vi "DCM Core Interface.vi"(6 "Device Inputs":dbl[](array[numeric]), 8 "error in":errorcluster, 9 "Device Outputs in":dbl[](array[numeric]), 10 "DCM Ref":refnum<class "DCM - RT.lvclass">, 11 "DCM Core in":T1={"FIFO Indexes"={"A Run State"=-1, "B Run State"=-1, "Read"={"Status"={"System ADC"={"AI 1 [V]"=0, "AI 2 [V]"=0, "AI 3 [V]"=0, "AI 4 [V]"=0, "AI 5 [V]"=0, "AI 6 [V]"=0, "AI 7 [V]"=0, "AI 8 [V]"=0, "AI 9 [V]"=0, "AI 10 [V]"=0, "AI 11 [V]"=0, "AI 12 [V]"=0, "Temp HH 1-6 [C]"=0, "Temp HH 7-12 [C]"=0, "Temp DI A [C]"=0, "Temp DI Zener A [C]"=0, "Temp DI B [C]"=0, "Temp DI Zener B [C]"=0, "Temp CPU [C]"=0, "Temp Fan Intake [C]"=0, "Temp Secondary A [C]"=0, "Temp Primary A [C]"=0, "Temp Boost B [C]"=0, "Primary Range [V]"=0, "Primary A1A2 [V]"=0, "Primary A3A4 [V]"=0, "Primary B3B4 [V]"=0, "Primary B1B2 [V]"=0, "Secondary A1A2 [V]"=0, "Secondary A3A4 [V]"=0, "Secondary B3B4 [V]"=0, "Secondary B1B2 [V]"=0, "Ext HV A [V]"=0, "Ext HV B [V]"=0, "FET Driver [V]"=0, "Fan [V]"=-1, "Battery [V]"=0, "DRVP [V]"=0, "Key [V]"=0, "DI Zener A [V]"=0, "DI Zener B [V]"=0, "Pump Zener A [V]"=0, "Pump Zener B [V]"=0, "MPRD [V]"=0}, "IO Lock"=0, "HH Mode Config Error"=0, "Fan Speed 1 [RPM]"=0, "Fan Speed 2 [RPM]"=0, "Firmware Major Rev"=0, "Firmware Minor Rev"=0, "Internal Fault"=-1, "Fault Value"=-1}, "A DI Faults"=[], "B DI Faults"=[], "HH Status"=[]}, "Write"={"A Config"={"PowerSupplyEnable"=0, "InjectEnable"=0, "BoostVoltage"=0}, "B Config"={"PowerSupplyEnable"=0, "InjectEnable"=0, "BoostVoltage"=0}, "HH Config"=[], "System Settings"={"MPRD"=0, "UserLED1"=0, "UserLED2"=0}, "A Fault Clear"={"1"=0, "2"=0, "3"=0, "4"=0, "5"=0, "6"=0, "7"=0, "8"=0}, "B Fault Clear"={"1"=0, "2"=0, "3"=0, "4"=0, "5"=0, "6"=0, "7"=0, "8"=0}}}, "Settings"={"A Configuration"={"Configuration"=enum."Solenoid Unipolar 4", "Power Supply Enable"=FALSE, "Boost Voltage [V]"=0.0, "Inject Enable"=FALSE, "DI Zener Enable"=FALSE, "DI Zener Voltage [V]"=0.0, "Pump Zener Enable"=FALSE, "Pump Zener Voltage [V]"=0.0, "Boost Clamp [V]"=0.0}, "B Configuration"={"Configuration"=enum."Solenoid Unipolar 4", "Power Supply Enable"=FALSE, "Boost Voltage [V]"=0.0, "Inject Enable"=FALSE, "DI Zener Enable"=FALSE, "DI Zener Voltage [V]"=0.0, "Pump Zener Enable"=FALSE, "Pump Zener Voltage [V]"=0.0, "Boost Clamp [V]"=0.0}, "System Settings"={"MPRD"=FALSE, "IO Lock MPRD Disable"=FALSE, "User LED 1"=enum."Off", "User LED 2"=enum."Off", "DI HS Fault Filter Time [s]"=0.0, "Clamp Fault Filter Time [s]"=0.0, "HH Shoot Through Time [s]"=0.0, "HH ISeq Dur PS"=0, "HH Open Threshold [A]"=0.0}}} {"Settings"."System Settings"."HH Open Threshold [A]" min=0 max=8 format="%#_3p"; "Settings"."System Settings"."HH ISeq Dur PS" items=["3.3ms @ 20MHz"=0, "6.5ms @ 10MHz"=4, "13ms @ 5MHz"=6, "26ms @ 2.5MHz"=7]; "Settings"."System Settings"."HH Shoot Through Time [s]" min=0 max=0.003277 format="%#_3p"; "Settings"."System Settings"."Clamp Fault Filter Time [s]" min=0 max=0.003277 format="%#_3p"; "Settings"."System Settings"."DI HS Fault Filter Time [s]" min=0 max=0.003277 format="%#_3p"; "Settings"."B Configuration"."Pump Zener Voltage [V]" min=0 max=240 format="%#_13g"; "Settings"."B Configuration"."DI Zener Voltage [V]" min=0 max=100 format="%#_13g"; "Settings"."B Configuration"."Boost Clamp [V]" min=0 max=220 format="%#_13g"; "Settings"."B Configuration"."Boost Voltage [V]" min=0 max=220 format="%#_13g"; "Settings"."A Configuration"."Pump Zener Voltage [V]" min=0 max=240 format="%#_13g"; "Settings"."A Configuration"."DI Zener Voltage [V]" min=0 max=100 format="%#_13g"; "Settings"."A Configuration"."Boost Clamp [V]" min=0 max=220 format="%#_13g"; "Settings"."A Configuration"."Boost Voltage [V]" min=0 max=220 format="%#_13g"; "FIFO Indexes"."Write"."HH Config"."ISeq"."Duration [s]" min=0 max=26; "FIFO Indexes"."Write"."HH Config"."ISeq"."Lower [A]" min=0 max=8; "FIFO Indexes"."Write"."HH Config"."ISeq"."Upper [A]" min=0 max=8}) -> (0 "error out":errorcluster, 1 "Device Outputs out":dbl[](array[numeric]))   [LabVIEW 2016, in "DCM Engine.lvlib"]
uses:
  DCM Engine.lvlib
  Shared/Types/DCM Core.ctl
  Shared/Types/System State Indexes.ctl
  Shared/Types/DI Faults Indexes.ctl
  Shared/Types/HH Status Indexes.ctl
  Shared/Types/HH Config Indexes.ctl
  <vilib>/Powertrain Controls/Device Drivers/DCM/Rev0/RT/Configuration.ctl
  <vilib>/Powertrain Controls/Device Drivers/DCM/Rev0/FPGA/DI - Bank Configuration.ctl
  <vilib>/Powertrain Controls/Device Drivers/DCM/Rev0/RT/System Settings.ctl
  <vilib>/Powertrain Controls/Device Drivers/DCM/Rev0/RT/User LED.ctl
  <vilib>/Powertrain Controls/Device Drivers/DCM/HH/RT/Duration Pre Scale.ctl
  Built/DCM Classes Packed/Pharlap/C/DCM-Classes.lvlibp/DCM/Rev0/RT/DCM - RT.lvclass
  DCM Shared.lvlib
  <vilib>/Powertrain Controls/Device Drivers/DCM/Rev0/RT/DCM - RT.lvclass
  <vilib>/Powertrain Controls/Device Drivers/DCM/Rev0/FPGA/DCM - FPGA.lvlib
  <vilib>/Powertrain Controls/Device Drivers/DCM/HH/RT/DCM - RT - HH.lvlib
panel:
  # "Voltage [DV]"
  # "Voltage [V]"
  # "Voltage [DV]"
  # "Voltage [V]"
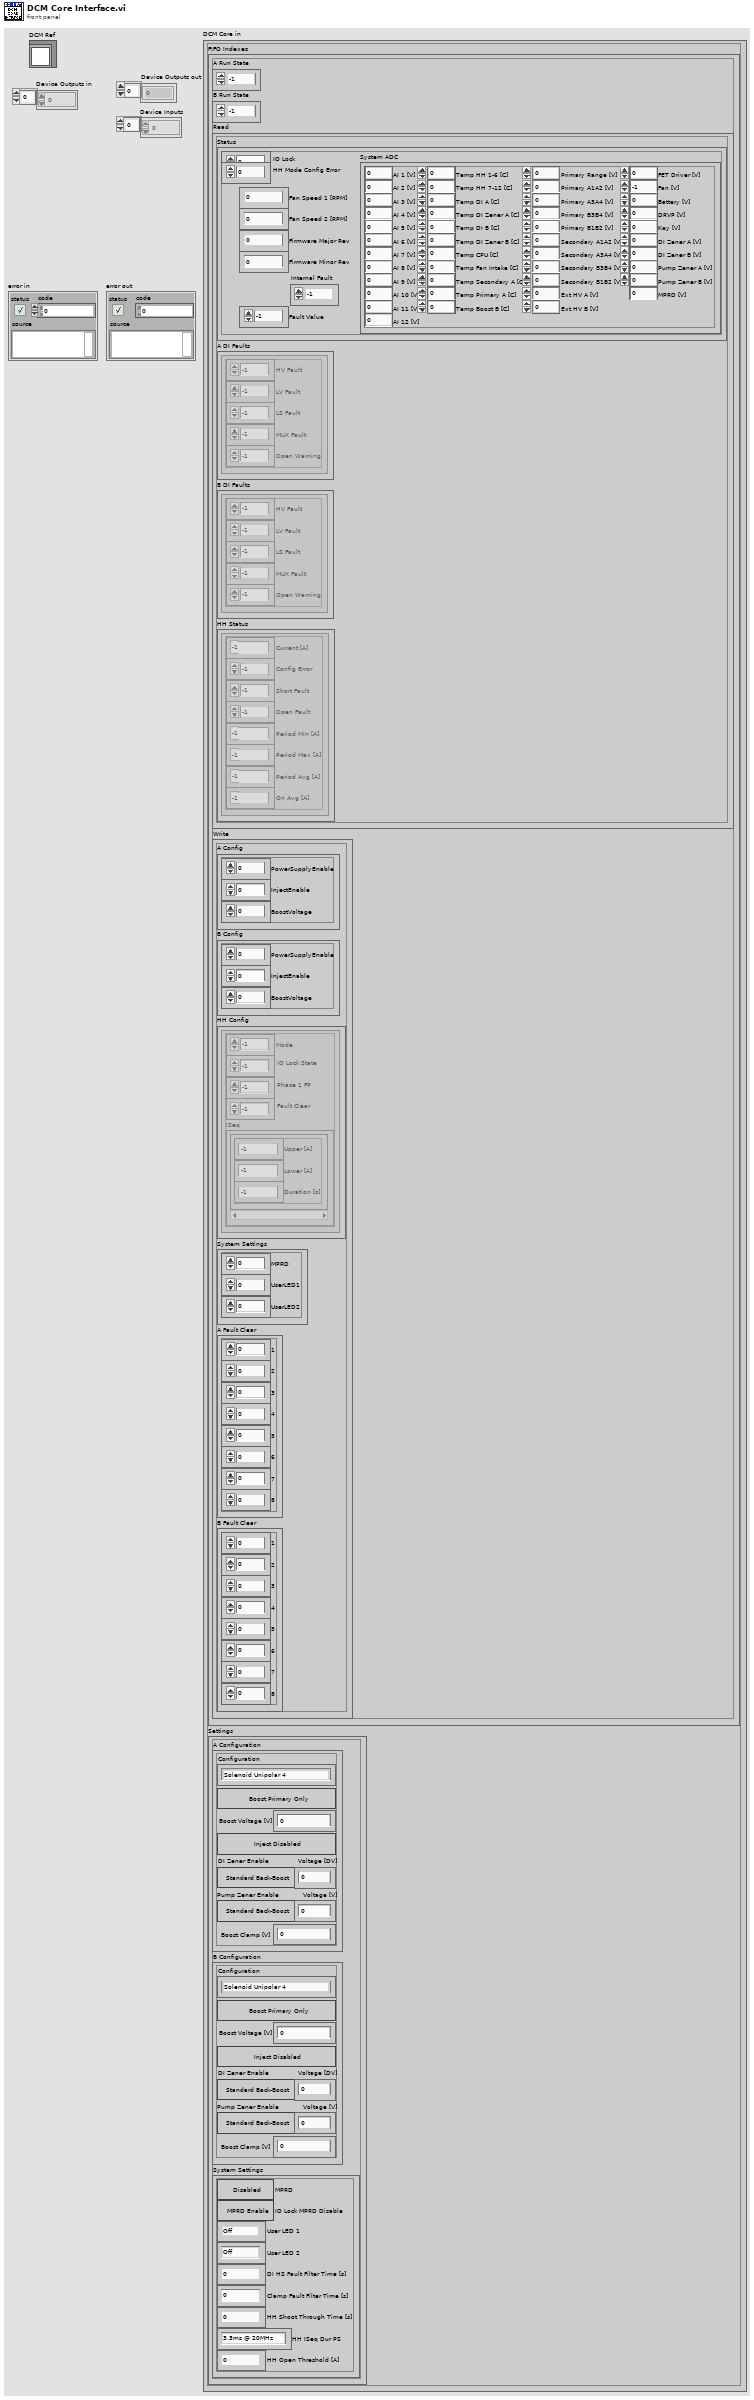
[diagram p1: front panel]
types:
  T1 = typedef "DCM Shared.lvlib/DCM Core.ctl" = cluster{"FIFO Indexes":cluster{"A Run State":i32, "B Run State":i32, "Read":cluster{"Status":T2, "A DI Faults":T3[], "B DI Faults":T3[], "HH Status":T4[]}, "Write":cluster{"A Config":cluster{"PowerSupplyEnable":i32, "InjectEnable":i32, "BoostVoltage":i32}, "B Config":cluster{"PowerSupplyEnable":i32, "InjectEnable":i32, "BoostVoltage":i32}, "HH Config":T5[], "System Settings":cluster{"MPRD":i32, "UserLED1":i32, "UserLED2":i32}, "A Fault Clear":cluster{"1":i32, "2":i32, "3":i32, "4":i32, "5":i32, "6":i32, "7":i32, "8":i32}, "B Fault Clear":cluster{"1":i32, "2":i32, "3":i32, "4":i32, "5":i32, "6":i32, "7":i32, "8":i32}}}, "Settings":cluster{"A Configuration":T6, "B Configuration":T6, "System Settings":T8}}
  T2 = typedef "DCM Shared.lvlib/System State Indexes.ctl" = cluster{"System ADC":cluster{"AI 1 [V]":i32, "AI 2 [V]":i32, "AI 3 [V]":i32, "AI 4 [V]":i32, "AI 5 [V]":i32, "AI 6 [V]":i32, "AI 7 [V]":i32, "AI 8 [V]":i32, "AI 9 [V]":i32, "AI 10 [V]":i32, "AI 11 [V]":i32, "AI 12 [V]":i32, "Temp HH 1-6 [C]":i32, "Temp HH 7-12 [C]":i32, "Temp DI A [C]":i32, "Temp DI Zener A [C]":i32, "Temp DI B [C]":i32, "Temp DI Zener B [C]":i32, "Temp CPU [C]":i32, "Temp Fan Intake [C]":i32, "Temp Secondary A [C]":i32, "Temp Primary A [C]":i32, "Temp Boost B [C]":i32, "Primary Range [V]":i32, "Primary A1A2 [V]":i32, "Primary A3A4 [V]":i32, "Primary B3B4 [V]":i32, "Primary B1B2 [V]":i32, "Secondary A1A2 [V]":i32, "Secondary A3A4 [V]":i32, "Secondary B3B4 [V]":i32, "Secondary B1B2 [V]":i32, "Ext HV A [V]":i32, "Ext HV B [V]":i32, "FET Driver [V]":i32, "Fan [V]":i32, "Battery [V]":i32, "DRVP [V]":i32, "Key [V]":i32, "DI Zener A [V]":i32, "DI Zener B [V]":i32, "Pump Zener A [V]":i32, "Pump Zener B [V]":i32, "MPRD [V]":i32}, "IO Lock":i32, "HH Mode Config Error":i32, "Fan Speed 1 [RPM]":i32, "Fan Speed 2 [RPM]":i32, "Firmware Major Rev":i32, "Firmware Minor Rev":i32, "Internal Fault":i32, "Fault Value":i32}
  T3 = typedef "DCM Shared.lvlib/DI Faults Indexes.ctl" = cluster{"HV Fault":i32, "LV Fault":i32, "LS Fault":i32, "MUX Fault":i32, "Open Warning":i32}
  T4 = typedef "DCM Shared.lvlib/HH Status Indexes.ctl" = cluster{"Current [A]":i32, "Config Error":i32, "Short Fault":i32, "Open Fault":i32, "Period Min [A]":i32, "Period Max [A]":i32, "Period Avg [A]":i32, "On Avg [A]":i32}
  T5 = typedef "DCM Shared.lvlib/HH Config Indexes.ctl" = cluster{"Mode":i32, "IO Lock State":i32, "Phase 1 FP":i32, "Fault Clear":i32, "ISeq":cluster{"Upper [A]":i32, "Lower [A]":i32, "Duration [s]":i32}[]}
  T6 = typedef "DCM - RT.lvclass/Configuration.ctl" = cluster{"Configuration":T7, "Power Supply Enable":bool, "Boost Voltage [V]":sgl, "Inject Enable":bool, "DI Zener Enable":bool, "DI Zener Voltage [V]":sgl, "Pump Zener Enable":bool, "Pump Zener Voltage [V]":sgl, "Boost Clamp [V]":sgl}
  T7 = typedef "DCM - FPGA.lvlib/DI - Bank Configuration.ctl" = enum8{"Solenoid Unipolar 4", "Solenoid Unipolar 7 (Muxed)", "Solenoid Unipolar 8 (Muxed)", "Solenoid Bipolar 2", "Solenoid Bipolar 3 (Muxed)", "Piezo Unipolar 2", "Piezo Unipolar 3 (Muxed)", "Piezo Unipolar 4 (Muxed)", "Piezo Bipolar 2", "Piezo Bipolar 3 (Muxed)"}
  T8 = typedef "DCM - RT.lvclass/System Settings.ctl" = cluster{"MPRD":bool, "IO Lock MPRD Disable":bool, "User LED 1":T9, "User LED 2":T9, "DI HS Fault Filter Time [s]":sgl, "Clamp Fault Filter Time [s]":sgl, "HH Shoot Through Time [s]":sgl, "HH ISeq Dur PS":T10, "HH Open Threshold [A]":sgl}
  T9 = typedef "DCM - RT.lvclass/User LED.ctl" = enum16{"Off", "Yellow", "Green"}
  T10 = typedef "DCM - RT - HH.lvlib/Duration Pre Scale.ctl" = u8
  T11 = typedef "DCM-Classes.lvlibp/DCM - RT.lvclass/System Settings.ctl" = cluster{"MPRD":bool, "IO Lock MPRD Disable":bool, "User LED 1":T12, "User LED 2":T12, "DI HS Fault Filter Time [s]":sgl, "Clamp Fault Filter Time [s]":sgl, "HH Shoot Through Time [s]":sgl, "HH ISeq Dur PS":T13, "HH Open Threshold [A]":sgl}
  T12 = typedef "DCM-Classes.lvlibp/DCM - RT.lvclass/User LED.ctl" = enum16{"Off", "Yellow", "Green"}
  T13 = typedef "DCM-Classes.lvlibp/DCM - RT - HH.lvlib/Duration Pre Scale.ctl" = u8
  T14 = typedef "DCM-Classes.lvlibp/DCM - RT.lvclass/Configuration.ctl" = cluster{"Configuration":T15, "Power Supply Enable":bool, "Boost Voltage [V]":sgl, "Inject Enable":bool, "DI Zener Enable":bool, "DI Zener Voltage [V]":sgl, "Pump Zener Enable":bool, "Pump Zener Voltage [V]":sgl, "Boost Clamp [V]":sgl}
  T15 = typedef "DCM-Classes.lvlibp/DCM - FPGA.lvlib/DI - Bank Configuration.ctl" = enum8{"Solenoid Unipolar 4", "Solenoid Unipolar 7 (Muxed)", "Solenoid Unipolar 8 (Muxed)", "Solenoid Bipolar 2", "Solenoid Bipolar 3 (Muxed)", "Piezo Unipolar 2", "Piezo Unipolar 3 (Muxed)", "Piezo Unipolar 4 (Muxed)", "Piezo Bipolar 2", "Piezo Bipolar 3 (Muxed)"}
  T16 = typedef "DCM - FPGA - Tools.lvlib/8 Channels.ctl" = cluster{"1":bool, "2":bool, "3":bool, "4":bool, "5":bool, "6":bool, "7":bool, "8":bool}
  T17 = typedef "DCM-Classes.lvlibp/DCM - RT - HH.lvlib/Config.ctl" = cluster{"Mode":T18, "IO Lock State":bool, "Phase 1 FP":bool, "Fault Clear":bool, "ISeq":T19[]}
  T18 = typedef "DCM-Classes.lvlibp/DCM - RT - HH.lvlib/Mode.ctl" = enum16{"Off", "Lowside", "Highside", "PFI", "Full H", "3-Phase"}
  T19 = typedef "DCM-Classes.lvlibp/DCM - RT - HH.lvlib/ISeq.ctl" = cluster{"Upper [A]":sgl, "Lower [A]":sgl, "Duration [s]":sgl}
  T20 = typedef "DCM-Classes.lvlibp/DCM - RT.lvclass/Run State.ctl" = enum8{"Idle", "Warmup", "Ready To Inject", "Cool Down"}
  T21 = typedef "DCM-Classes.lvlibp/DCM - RT.lvclass/System State.ctl" = cluster{"System ADC":T22, "IO Lock":bool, "HH Mode Config Error":bool, "Fan Speed 1 [RPM]":sgl, "Fan Speed 2 [RPM]":sgl, "Firmware Major Rev":u16, "Firmware Minor Rev":u16, "Internal Fault":T23, "Fault Value":dbl}
  T22 = typedef "DCM-Classes.lvlibp/DCM - RT.lvclass/System ADC.ctl" = cluster{"AI 1 [V]":sgl, "AI 2 [V]":sgl, "AI 3 [V]":sgl, "AI 4 [V]":sgl, "AI 5 [V]":sgl, "AI 6 [V]":sgl, "AI 7 [V]":sgl, "AI 8 [V]":sgl, "AI 9 [V]":sgl, "AI 10 [V]":sgl, "AI 11 [V]":sgl, "AI 12 [V]":sgl, "Temp HH 1-6 [C]":sgl, "Temp HH 7-12 [C]":sgl, "Temp DI A [C]":sgl, "Temp DI Zener A [C]":sgl, "Temp DI B [C]":sgl, "Temp DI Zener B [C]":sgl, "Temp CPU [C]":sgl, "Temp Fan Intake [C]":sgl, "Temp Secondary A [C]":sgl, "Temp Primary A [C]":sgl, "Temp Boost B [C]":sgl, "Primary Range [V]":sgl, "Primary A1A2 [V]":sgl, "Primary A3A4 [V]":sgl, "Primary B3B4 [V]":sgl, "Primary B1B2 [V]":sgl, "Secondary A1A2 [V]":sgl, "Secondary A3A4 [V]":sgl, "Secondary B3B4 [V]":sgl, "Secondary B1B2 [V]":sgl, "Ext HV A [V]":sgl, "Ext HV B [V]":sgl, "FET Driver [V]":sgl, "Fan [V]":sgl, "Battery [V]":sgl, "DRVP [V]":sgl, "Key [V]":sgl, "DI Zener A [V]":sgl, "DI Zener B [V]":sgl, "Pump Zener A [V]":sgl, "Pump Zener B [V]":sgl, "MPRD [V]":sgl}
  T23 = typedef "DCM-Classes.lvlibp/DCM - RT.lvclass/Internal Fault.ctl" = enum32{"None", "Temp HH 1-6", "Temp HH 7-12", "Temp DI A", "Temp DI Zener A", "Temp DI B", "Temp DI Zener B", "Temp Intake", "Temp Primary A", "Temp Secondary A", "Temp Boost B", "Temp CPU", "Low Battery", "Inrush Protection", "A Run Enable", "B Run Enable"}
  T24 = typedef "DCM-Classes.lvlibp/DCM - FPGA.lvlib/DI - Faults.ctl" = cluster{"HV Fault":bool, "LV Fault":bool, "LS Fault":bool, "MUX Fault":bool, "Open Warning":bool}
  T25 = typedef "DCM-Classes.lvlibp/DCM - RT - HH.lvlib/Status.ctl" = cluster{"Current [A]":sgl, "Config Error":bool, "Short Fault":bool, "Open Fault":bool, "Period Min [A]":sgl, "Period Max [A]":sgl, "Period Avg [A]":sgl, "On Avg [A]":sgl}
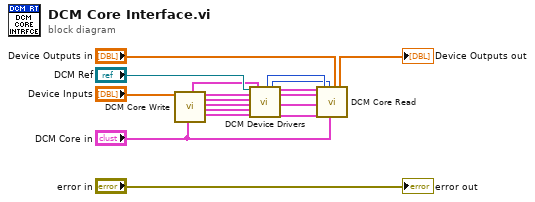
[diagram p0: block diagram]
diagram:
  n1 = call "DCM Core Write.vi"("Device Inputs"="Device Inputs", "DCM Core in"="DCM Core in") -> ("System Settings out"=w13:T11, "A Configuration"=w6:T14, "A Fault Clear out"=w10:T16, "B Configuration"=w9:T14, "B Fault Clear out"=w12:T16, "HH Config"=w8:T17[])  [unwired: 12 in]
  n2 = call-dynamic "DCM Device Drivers.vi"("DCM Reference"="DCM Ref", "A Configuration"=w6, "A Fault Clear"=w10, "B Configuration"=w9, "B Fault Clear"=w12, "HH Config"=w8, "System Settings"=w13) -> ("A Run State"=w2:T20, "B Run State"=w1:T20, "System State"=w11:T21, "A DI Faults"=w3:T24[], "B DI Faults"=w7:T24[], "HH Status"=w14:T25[])  [unwired: 4 in, 3 out]
  n3 = call "DCM Core Read.vi"("System State"=w11, "A DI Faults"=w3, "B DI Faults"=w7, "HH Status"=w14, "A Run State"=w2, "B Run State"=w1, "DCM Core in"="DCM Core in", "Device Outputs in"="Device Outputs in") -> ("Device Outputs out"=→"Device Outputs out":dbl[])  [unwired: 11 in]
  "error out" <- "error in"
